vi "Pre Install Script.vi"() -> ()   [LabVIEW 2013]
uses:
  <vilib>/Utility/sysdir.llb/System Directory Type.ctl
panel:
  out "error out":errorcluster
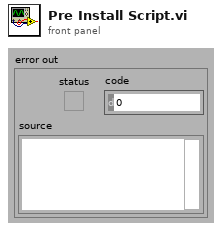
[diagram p1: front panel]
types:
  T1 = typedef "System Directory Type.ctl" = i32
  T2 = enum16{"open", "replace", "create", "open or create", "replace or create", "replace or create with confirmation"}
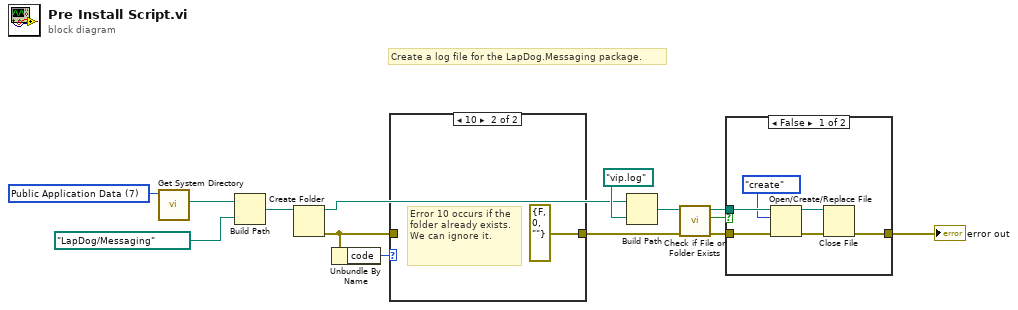
[diagram p0: block diagram]
diagram:
  w14 = T1 7 items=["User Home", "User Desktop", "User Documents", "User Application Data", "User Preferences", "User Temporary", "Public Documents", "Public Application Data", "Public Preferences", "System Core Libraries", "System Installed Libraries", "Application Files", "Boot Volume Root"] ("system directory type")
  # "Create a log file for the LapDog.Messaging package."
  n1 = call <vilib>:"Get System Directory.vi"("system directory type"=w14) -> ("system directory"=w13:path)  [unwired: 10 in]
  n2 = Build Path(base path=w13, name or relative path=path "LapDog/Messaging" ("Log File Path")) -> (appended path=w11:path)
  n3 = Create Folder(path (use dialog)=w11) -> (created path=w6:path, error out=w9:errorcluster)  [unwired: 2 in, 1 out]
  n4 = Unbundle By Name(w9) -> ("code"=w10:i32)
  n5 = case shown="10" w10 {
    tunnel: w9 -> [w15 _]
    tunnel: [w15 errorcluster {"status"=FALSE, "code"=0, "source"=""} ("error out")] -> w7
    frame Default {
    }
    frame 10 {
      # "Error 10 occurs if the folder already exists.  We can ignore it."
    }
  }
  n6 = Build Path(base path=w6, name or relative path=path "vip.log" ("Log File Path")) -> (appended path=w5:path)
  n7 = call <vilib>:"Check if File or Folder Exists.vi"("error in (no error)"=w7, "path"=w5) -> ("error out"=w3:errorcluster, "file or folder exists?"=w4:bool, "dup path"=w2:path)  [unwired: 7 in]
  n8 = case shown="False" w4 {
    tunnel: w3 -> [w22 w23]
    tunnel: w2 -> [w21 _]
    tunnel: [w17 w23] -> w1
    frame False {
      n9 = Open/Create/Replace File(file path (use dialog)=w21, error in=w22, operation (0:open)=T2."create") -> (refnum out=w19:refnum<file>, error out=w18:errorcluster)  [unwired: 3 in, 1 out]
      n10 = Close File(refnum=w19, error in=w18) -> (error out=w17:errorcluster)  [unwired: 1 out]
    }
    frame True {
    }
  }
  "error out" <- w1
